vi "Blendingsubvi.vi"() -> (3 "index of element":i32)   [LabVIEW 2021]
uses:
  <vilib>/numeric/Random Number (Range) U64.vi
  <vilib>/numeric/sub_Random U32.vi
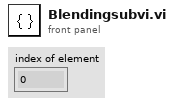
[diagram p1: front panel]
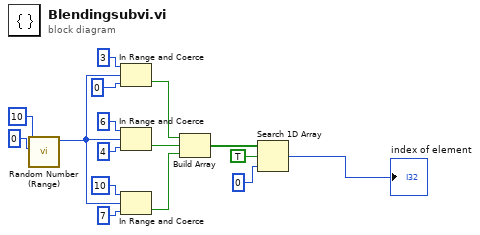
[diagram p0: block diagram]
diagram:
  n1 = call-poly <vilib>:"Random Number (Range).vi"("lower bound (0)"=u64 0, "upper bound (100)"=u64 10) -> ("number"=w5:u64)  [unwired: 9 in]
  n2 = In Range and Coerce(upper limit=u64 3, x=w5, lower limit=u64 0) -> (In Range?=w11:bool)  [unwired: 1 out]
  n3 = In Range and Coerce(upper limit=u64 6, x=w5, lower limit=u64 4) -> (In Range?=w12:bool)  [unwired: 1 out]
  n4 = In Range and Coerce(upper limit=u64 10, x=w5, lower limit=u64 7) -> (In Range?=w13:bool)  [unwired: 1 out]
  n5 = Build Array(w11, w12, w13) -> (w10:bool[])
  n6 = Search 1D Array(1D array=w10, element=TRUE, start index (0)=0) -> (index of element=→"index of element":i32)
